vi "量程转换.vi"(1 "输入":i32[](array[numeric]), 2 "量程输入":i32(ring) items=["±10000mV", "±5000mV", "±2500mV", "0-10000mV", "0-5000mV"]) -> (0 "输出":dbl[](array[numeric]))   [LabVIEW 2012]
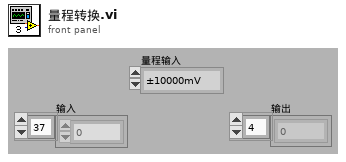
[diagram p1: front panel]
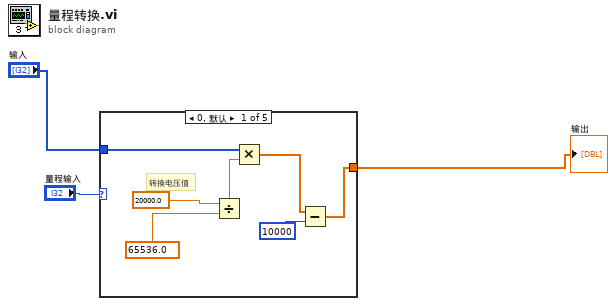
[diagram p0: block diagram]
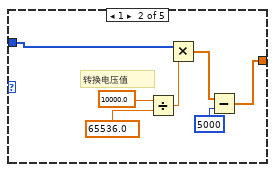
[diagram p2: hidden frame]
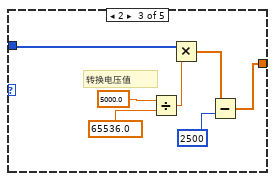
[diagram p3: hidden frame]
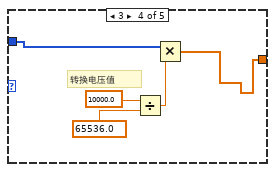
[diagram p4: hidden frame]
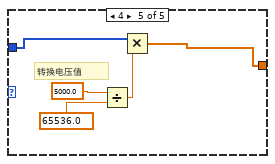
[diagram p5: hidden frame]
diagram:
  n1 = case shown="0, 默认" "量程输入" {
    tunnel: "输入" -> [w7 w11 w18 w25 w30]
    tunnel: [w5 w14 w19 w26 w31] -> w1
    frame 0, Default {
      # "转换电压值"
      n2 = Divide(x=20000.0, y=65536.0) -> (x/y=w8:dbl)
      n3 = Multiply(x=w7, y=w8) -> (x*y=w6:dbl[])
      n4 = Subtract(x=w6, y=10000) -> (x-y=w5:dbl[])
    }
    frame 1 {
      # "转换电压值"
      n5 = Divide(x=10000.0, y=65536.0) -> (x/y=w15:dbl)
      n6 = Multiply(x=w11, y=w15) -> (x*y=w13:dbl[])
      n7 = Subtract(x=w13, y=5000) -> (x-y=w14:dbl[])
    }
    frame 2 {
      # "转换电压值"
      n8 = Divide(x=5000.0, y=65536.0) -> (x/y=w21:dbl)
      n9 = Multiply(x=w18, y=w21) -> (x*y=w20:dbl[])
      n10 = Subtract(x=w20, y=2500) -> (x-y=w19:dbl[])
    }
    frame 3 {
      # "转换电压值"
      n11 = Divide(x=10000.0, y=65536.0) -> (x/y=w27:dbl)
      n12 = Multiply(x=w25, y=w27) -> (x*y=w26:dbl[])
    }
    frame 4 {
      # "转换电压值"
      n13 = Divide(x=5000.0, y=65536.0) -> (x/y=w32:dbl)
      n14 = Multiply(x=w30, y=w32) -> (x*y=w31:dbl[])
    }
  }
  "输出" <- w1
